vi "Ensure window is completely visible on screen.vi"(8 "error in (no error)":errorcluster, 11 "VI Refnum":refnum<vi>) -> (0 "error out":errorcluster)   [LabVIEW 2011, in "COSYLib.lvlib"]
uses:
  COSYLib.lvlib
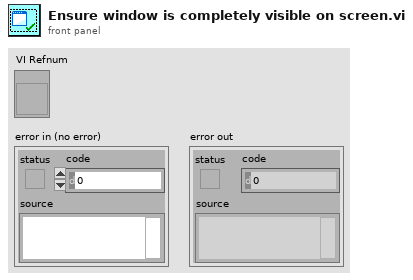
[diagram p1: front panel]
types:
  T1 = typedef "LVRectTypeDef.ctl" = cluster{"left":i16, "top":i16, "right":i16, "bottom":i16}
  T2 = typedef "LVAllMonitorsDisplayTypeDef.ctl" = cluster{"Bounds":cluster{"Left":i16, "Top":i16, "Right":i16, "Bottom":i16}, "Depth":i16}[]
  T3 = cluster{"Left":i16, "Top":i16, "Right":i16, "Bottom":i16}
  T4 = cluster{"left":i16, "top":i16, "right":i16, "bottom":i16}
  T5 = cluster{i32, "Bounds":cluster{"Left":i16, "Top":i16, "Right":i16, "Bottom":i16}}
  T6 = cluster{i32, "Bounds":cluster{"Left":i16, "Top":i16, "Right":i16, "Bottom":i16}}[]
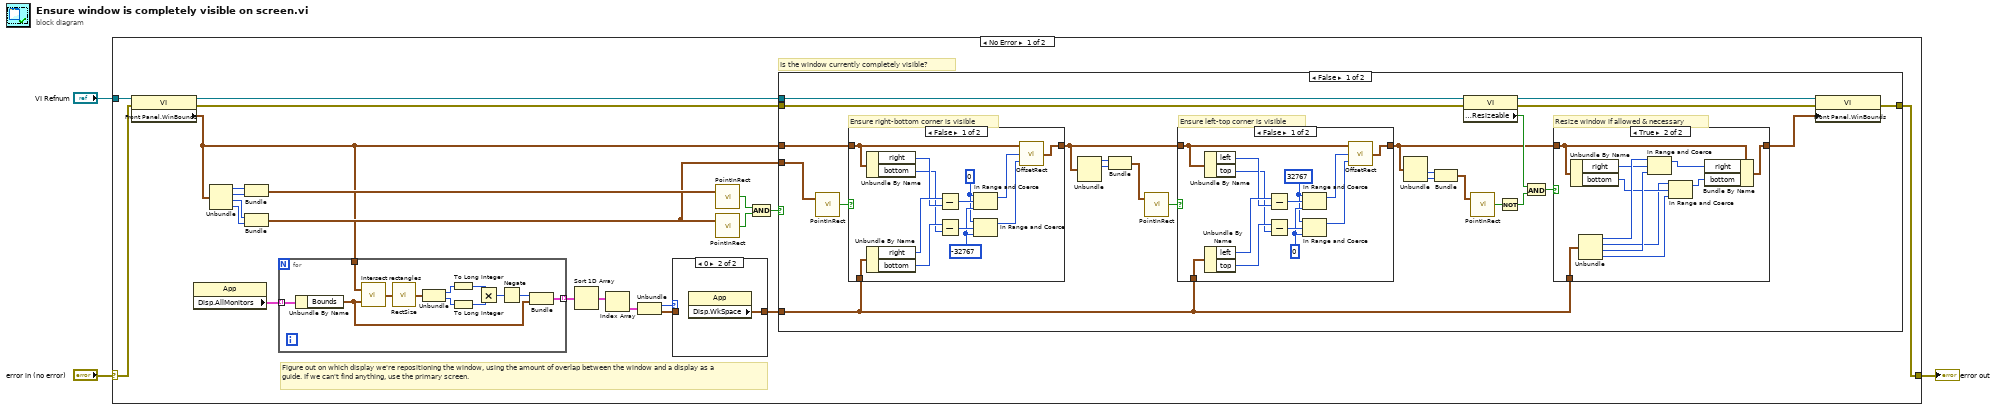
[diagram p0: block diagram]
diagram:
  n1 = case shown="No Error" "error in (no error)" {
    selector: "error in (no error)" -> [w6 w104]
    tunnel: "VI Refnum" -> [w25 _]
    tunnel: [w4 w104] -> w1
    frame No Error {
      # "Is the window currently completely visible?"
      # "Figure out on which display we're repositioning the window, using the amount of overlap between the window and a display as a guide. If we can't find anything, use the primary screen."
      n2 = property class="VI"(reference=w25, error in=w6) -> (reference out=w16:refnum<vi>, error out=w5:errorcluster, "Front Panel.WinBounds"=w13:T1)
      n3 = property class="App"() -> ("Disp.AllMonitors"=w14:T2)  [unwired: 2 in, 2 out]
      n4 = Unbundle(w13) -> ("left"=w24:i16, "top"=w23:i16, "right"=w22:i16, "bottom"=w21:i16)
      n5 = Bundle("left"=w24, "top"=w23) -> (w17:cluster{"left":i16, "top":i16})  [unwired: 1 in]
      n6 = Bundle("right"=w22, "bottom"=w21) -> (w15:cluster{"right":i16, "bottom":i16})  [unwired: 1 in]
      n7 = for {
        tunnel: w14 -> [w39] mode=indexing
        tunnel: w13 -> [w38]
        tunnel: [w34] -> w12 mode=indexing
        n8 = Unbundle By Name(w39) -> ("Bounds"=w35:T3)
        n9 = call "Intersect rectangles.vi"("rect 2"=w35, "rect"=w38) -> ("intersection rect"=w31:T4)
        n10 = call <vilib>:"RectSize.vi"("rect"=w31) -> ("point"=w30:cluster{"x":i16, "y":i16})
        n11 = Unbundle(w30) -> ("x"=w37:i16, "y"=w36:i16)
        n12 = To Long Integer(number=w37) -> (32bit integer=w29:i32)
        n13 = To Long Integer(number=w36) -> (32bit integer=w28:i32)
        n14 = Multiply(x=w29, y=w28) -> (x*y=w32:i32)
        n15 = Negate(x=w32) -> (-x=w33:i32)
        n16 = Bundle(w33, "Bounds"=w35) -> (w34:T5)  [unwired: 1 in]
      }
      n17 = Sort 1D Array(array=w12) -> (sorted array=w11:T6)
      n18 = Index Array(array=w11) -> (element=w10:T5)  [unwired: 1 in]
      n19 = Unbundle(w10) -> (w9:i32, "Bounds"=w8:T3)
      n20 = case shown="0" w9 {
        tunnel: w8 -> [w26 _]
        tunnel: [w26 w27] -> w7
        frame Default {
        }
        frame 0 {
          n21 = property class="App"() -> ("Disp.WkSpace"=w27:T1)  [unwired: 2 in, 2 out]
        }
      }
      n22 = call <vilib>:"PointInRect.vi"("point"=w17) -> ("pt in rect"=w20:bool)  [unwired: 1 in]
      n23 = call <vilib>:"PointInRect.vi"("point"=w15) -> ("pt in rect"=w19:bool)  [unwired: 1 in]
      n24 = And(x=w20, y=w19) -> (x .and. y?=w18:bool)
      n25 = case shown="False" w18 {
        tunnel: w15 -> [w62 _]
        tunnel: w16 -> [w54 _]
        tunnel: w13 -> [w60 _]
        tunnel: w7 -> [w44 _]
        tunnel: w5 -> [w42 w103]
        tunnel: [w40 w103] -> w4
        frame False {
          # "Resize window if allowed & necessary"
          # "Ensure left-top corner is visible"
          # "Ensure right-bottom corner is visible"
          n26 = call <vilib>:"PointInRect.vi"("point"=w62) -> ("pt in rect"=w61:bool)  [unwired: 1 in]
          n27 = case shown="False" w61 {
            tunnel: w60 -> [w93 w102]
            tunnel: [w90 w102] -> w56
            tunnel: w44 -> [w89 _]
            frame False {
              w94 = i16 0 ("upper limit")
              w95 = i16 -32767 ("lower limit")
              n28 = Unbundle By Name(w93) -> ("right"=w100:i16, "bottom"=w98:i16)
              n29 = Unbundle By Name(w89) -> ("right"=w101:i16, "bottom"=w99:i16)
              n30 = Subtract(x=w101, y=w100) -> (x-y=w97:i16)
              n31 = Subtract(x=w99, y=w98) -> (x-y=w96:i16)
              n32 = In Range and Coerce(upper limit=w94, x=w97, lower limit=w95) -> (coerced(x)=w92:i16)  [unwired: 1 out]
              n33 = In Range and Coerce(upper limit=w94, x=w96, lower limit=w95) -> (coerced(x)=w91:i16)  [unwired: 1 out]
              n34 = call <vilib>:"OffsetRect.vi"("v"=w91, "h"=w92, "rect"=w93) -> ("offset rect"=w90:T4)
            }
            frame True {
            }
          }
          n35 = Unbundle(w56) -> ("left"=w59:i16, "top"=w58:i16)  [unwired: 2 out]
          n36 = Bundle("left"=w59, "top"=w58) -> (w57:cluster{"left":i16, "top":i16})  [unwired: 1 in]
          n37 = call <vilib>:"PointInRect.vi"("point"=w57) -> ("pt in rect"=w55:bool)  [unwired: 1 in]
          n38 = case shown="False" w55 {
            tunnel: w56 -> [w79 w88]
            tunnel: [w76 w88] -> w45
            tunnel: w44 -> [w75 _]
            frame False {
              w80 = i16 32767 ("upper limit")
              w81 = i16 0 ("lower limit")
              n39 = Unbundle By Name(w79) -> ("left"=w86:i16, "top"=w84:i16)
              n40 = Unbundle By Name(w75) -> ("left"=w87:i16, "top"=w85:i16)
              n41 = Subtract(x=w87, y=w86) -> (x-y=w83:i16)
              n42 = Subtract(x=w85, y=w84) -> (x-y=w82:i16)
              n43 = In Range and Coerce(upper limit=w80, x=w83, lower limit=w81) -> (coerced(x)=w78:i16)  [unwired: 1 out]
              n44 = In Range and Coerce(upper limit=w80, x=w82, lower limit=w81) -> (coerced(x)=w77:i16)  [unwired: 1 out]
              n45 = call <vilib>:"OffsetRect.vi"("v"=w77, "h"=w78, "rect"=w79) -> ("offset rect"=w76:T4)
            }
            frame True {
            }
          }
          n46 = Unbundle(w45) -> ("right"=w50:i16, "bottom"=w51:i16)  [unwired: 2 out]
          n47 = Bundle("right"=w50, "bottom"=w51) -> (w52:cluster{"right":i16, "bottom":i16})  [unwired: 1 in]
          n48 = property class="VI"(reference=w54, error in=w42) -> (reference out=w53:refnum<vi>, error out=w41:errorcluster, "Front Panel.Resizeable"=w48:bool)
          n49 = call <vilib>:"PointInRect.vi"("point"=w52) -> ("pt in rect"=w49:bool)  [unwired: 1 in]
          n50 = Not(x=w49) -> (.not. x?=w47:bool)
          n51 = And(x=w48, y=w47) -> (x .and. y?=w46:bool)
          n52 = case shown="True" w46 {
            tunnel: w45 -> [w63 w74]
            tunnel: [w63 w73] -> w43
            tunnel: w44 -> [_ w72]
            frame False {
            }
            frame True {
              n53 = Unbundle By Name(w74) -> ("right"=w69:i16, "bottom"=w66:i16)
              n54 = Unbundle(w72) -> ("left"=w71:i16, "top"=w65:i16, "right"=w70:i16, "bottom"=w64:i16)
              n55 = In Range and Coerce(upper limit=w71, x=w69, lower limit=w70) -> (coerced(x)=w68:i16)  [unwired: 1 out]
              n56 = In Range and Coerce(upper limit=w65, x=w66, lower limit=w64) -> (coerced(x)=w67:i16)  [unwired: 1 out]
              n57 = Bundle By Name(cluster=w74, "right"=w68, "bottom"=w67) -> (w73:T1)
            }
          }
          n58 = property class="VI"(reference=w53, error in=w41, "Front Panel.WinBounds"=w43) -> (error out=w40:errorcluster)  [unwired: 1 out]
        }
        frame True {
          # "Nothing to do: window is already completely visible :)"
        }
      }
    }
    frame Error {
    }
  }
  "error out" <- w1
